vi "Clone Template Actor.vi"(8 "error in (no error)":errorcluster, 11 "Destination Directory":path) -> (0 "error out":errorcluster, 2 "New Class Path":path)   [LabVIEW 2018, in "Scripting.lvlib"]
uses:
  Scripting.lvlib
  Templating-Root.vi
  Tooling-Root.vi
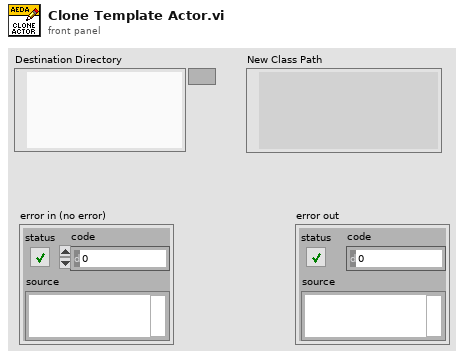
[diagram p1: front panel]
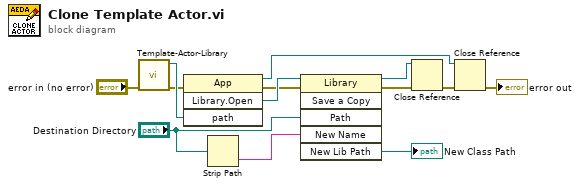
[diagram p0: block diagram]
diagram:
  n1 = call "Template-Actor-Library.vi"("error in (no error)"="error in (no error)") -> ("error out"=w12:errorcluster, "Template-Actor-Root"=w13:path)  [unwired: 9 in]
  n2 = invoke class="App" method="Library.Open"(error in=w12, "path"=w13) -> (reference out=w4:refnum<vi>, error out=w7:errorcluster, "Open Library"=w10:refnum<vi>)  [unwired: 2 in, 1 out]
  n3 = Strip Path(path="Destination Directory") -> (name=w8:string)  [unwired: 1 out]
  n4 = invoke class="Library" method="Save a Copy"(reference=w10, error in=w7, "Path"="Destination Directory", "New Name"=w8) -> (reference out=w6:refnum<vi>, error out=w2:errorcluster, "New Lib Path"=→"New Class Path":path)  [unwired: 2 in, 3 out]
  n5 = Close Reference(reference=w6, error in (no error)=w2) -> (error out=w5:errorcluster)
  n6 = Close Reference(reference=w4, error in (no error)=w5) -> (error out=→"error out":errorcluster)
